vi "输入数据解析.vi"(0 "单个参数补充":dbl, 1 "从板号":dbl=1.0, 2 "主板二维码":string="BNET01", 3 "从板二维码":string="BNET01", 5 "主板引用":refnum<vi>, 7 "从板引用":refnum<vi>, 9 "主板选项":string="三级故障阀值", 11 "枚举":enum16{"主板", "从板"}(ring), 12 "快换":bool caption="快换写入") -> (4 "输出数组":dbl[][](array[numeric]), 6 "数组长度":dbl[](array[numeric]), 8 "循环次数":i32, 10 "命令":u32, 14 "名称":string[](array[string]), 15 "命令序号":u32[](array[numeric]))   [LabVIEW 2013]
panel:
  out "从板信息":T1
  out "主板数据":T2
  out "低位子数组 18":i32[](array[numeric])
  out "低位子数组 17":i32[](array[numeric])
  out "低位子数组 16":i32[](array[numeric])
  out "低位子数组 15":i32[](array[numeric])
  out "低位子数组 14":i32[](array[numeric])
  out "低位子数组 13":i32[](array[numeric])
  out "低位子数组 12":i32[](array[numeric])
  out "低位子数组 11":i32[](array[numeric])
  out "低位子数组 10":i32[](array[numeric])
  out "低位子数组 9":i32[](array[numeric])
  out "低位子数组 8":i32[](array[numeric])
  out "低位子数组 7":i32[](array[numeric])
  out "低位子数组 6":i32[](array[numeric])
  out "低位子数组 5":i32[](array[numeric])
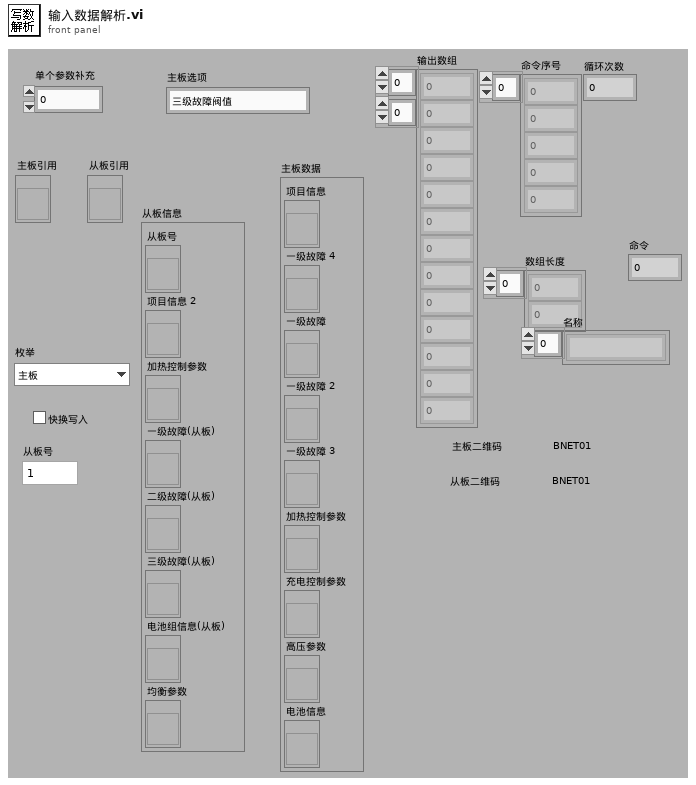
[diagram p1: front panel]
types:
  T1 = cluster{"从板号":refnum<vi>, "项目信息 2":refnum<vi>, "加热控制参数":refnum<vi>, "一级故障(从板)":refnum<vi>, "二级故障(从板)":refnum<vi>, "三级故障(从板)":refnum<vi>, "电池组信息(从板)":refnum<vi>, "均衡参数":refnum<vi>}
  T2 = cluster{"项目信息":refnum<vi>, "一级故障 4":refnum<vi>, "一级故障":refnum<vi>, "一级故障 2":refnum<vi>, "一级故障 3":refnum<vi>, "加热控制参数":refnum<vi>, "充电控制参数":refnum<vi>, "高压参数":refnum<vi>, "电池信息":refnum<vi>}
  T3 = cluster{"电池额定容量(A)":dbl, "使用者":dbl, "电池实际容量(A)":dbl, "车架(牌)号":string, "配置文件版本":string, "SOH(%)":dbl, "SOC(%)":dbl, "产品编号":string, "系统时钟":string}
  T4 = cluster{"总电压过高":dbl, "整组电压不均衡":dbl, "SOC过高":dbl, "单体电压过高":dbl, "总电压过低":dbl, "温度过高":dbl, "温度过低":dbl, "单组电压不均衡":dbl, "整组温度不均衡":dbl, "单组温度不均衡":dbl, "单体电压过低":dbl, "充电电流过高":dbl, "放电电流过高":dbl, "SOC过低":dbl, "内阻过大":dbl, "极柱温度过高":dbl, "SOH过低":dbl}
  T5 = cluster{"风机开启温度":dbl, "风机关闭温度":dbl, "加热开启温度":dbl, "加热关闭温度":dbl, "风机开启温差":dbl, "风机关闭温差":dbl, "加热关闭温差":dbl}
  T6 = cluster{"最大允许单体电压":dbl, "最大允许总电压":dbl, "最小允许单体电压":dbl, "最大允许充电电流":dbl, "最小允许充电电流":dbl, "最大允许充电温度":dbl, "最小允许充电温度":dbl, "电流步长":dbl}
  T7 = cluster{"电池串联":dbl, "电池并联":dbl, "累计放电总安时":dbl, "电池包额定容量":dbl, "电池包额定能量":dbl, "电池包额定总电压":dbl, "累计充电总安时":dbl, "电池充满次数":dbl, "电池放空次数":dbl, "电池充电次数":dbl, "电池生产日期":string, "电池厂家":string, "电池类型":string, "电池包组号":string, "电池包产权标识":string, "电池应用车型":string, "实际容量":dbl}
  T8 = cluster{"电压过高":dbl, "电压过低":dbl, "温度过高":dbl, "温度过低":dbl, "电压不均衡(V)":dbl, "温度不均衡":dbl, "SOC过低":dbl}
  T9 = cluster{"串联数":dbl, "并联数":dbl, "电池厂家":dbl, "电池类型":dbl, "额定能量":dbl, "额定容量":dbl, "实际容量":dbl, "额定总压":dbl, "产权标识":dbl, "应用车型":dbl, "电池包组号":dbl, "SOC":dbl, "充电总安时":dbl, "放电总这时":dbl, "放空次数":dbl, "充满次数":dbl, "充电次数":dbl, "车牌号":string, "生产日期":string, "最大允许单体电压":dbl, "最大允许总电压":dbl, "最大允许温度":dbl, "最小允许温度":dbl, "最大允许充电电流":dbl, "最小允许充电电流":dbl, "最小允许单体电压":dbl, "电流步长":dbl, "电池包序号":dbl}
  T10 = cluster{"充电结束电压(90%)":sgl, "充电结束电压(91%)":sgl, "充电结束电压(92%)":sgl, "充电结束电压(93%)":sgl, "充电结束电压(94%)":sgl, "均衡计算-电压高阀值1级":sgl, "均衡计算-电压高阀值2级":sgl, "均衡计算-电压低阀值1级":sgl, "均衡计算-电压低阀值2级":sgl, "均衡计算-最低电压阀值":sgl, "均衡停止-最低电压阀值":sgl, "均衡计算-电压极差阀值":sgl, "充电结束电压(95%)":sgl, "充电结束电压(96%)":sgl, "充电结束电压(97%)":sgl, "充电结束电压(98%)":sgl, "充电结束电压(99%)":sgl, "充电结束电压(100%)":sgl}
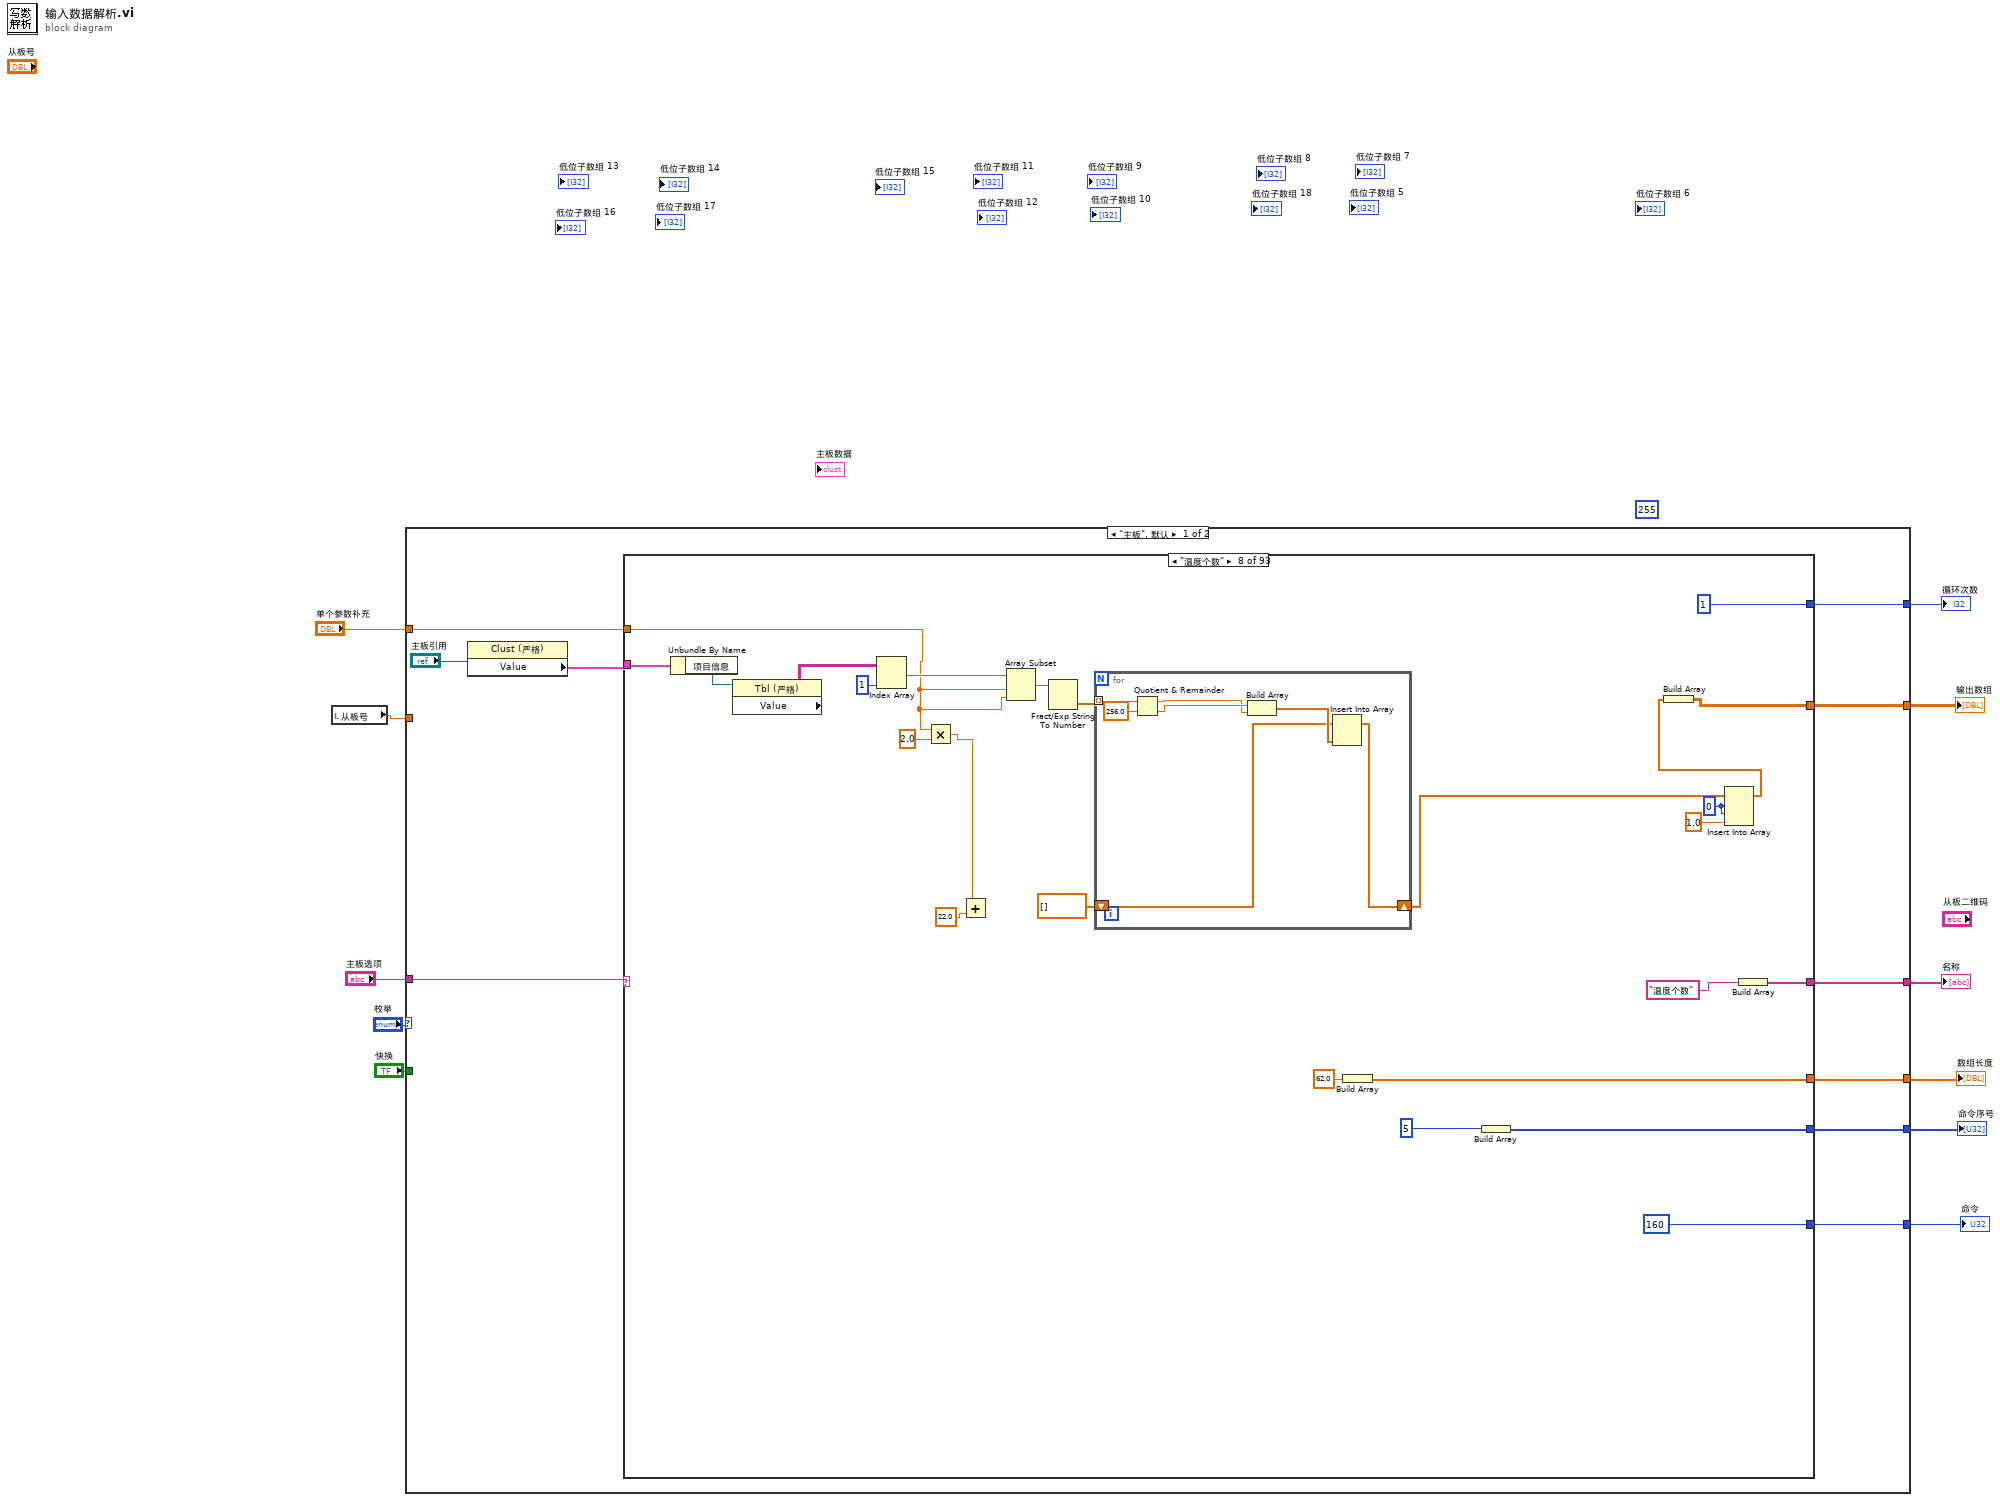
[diagram p0: block diagram]
diagram:
  (unwired) 255 ("高字节1")
  n1 = local read "从板号"() -> (w3:dbl)
  n2 = case shown="\"主板\", 默认" "枚举" {
    tunnel: "主板选项" -> [w21 w14879]
    tunnel: "单个参数补充" -> [w20 w14874]
    tunnel: [w19 w14878] -> w9
    tunnel: [w18 w14876] -> w8
    tunnel: [w17 w14875] -> w7
    tunnel: [w16 w14877] -> w6
    tunnel: "快换" -> [_ w14873]
    tunnel: w3 -> [_ w14872]
    tunnel: [w13 w14869] -> w2
    tunnel: [w12 w14868] -> w1
    frame "主板", Default {
      n3 = property class="Clust (严格)"(reference="主板引用") -> ("Value"=w14:T2)  [unwired: 1 in, 2 out]
      n4 = case shown="\"温度个数\"" w21 {
        tunnel: w20 -> [w29 w290 _ _ w576 w605 w636 w658 w696 _ _ _ _ _ _ _ _ _ _ _ _ _ _ _ _ _ _ _ _ _ _ _ _ _ _ _ _ _ _ _ _ _ _ _ _ _ _ _ _ _ _ _ _ _ _ _ _ _ _ _ _ _ _ _ _ _ _ _ _ _ _ _ _ _ _ _ _ _ _ _ _ _ _ _ _ _ _ _ _ _ _ _ _]
        tunnel: w14 -> [w27 w288 w549 _ w589 w622 w649 w678 w709 w737 w774 w789 w813 _ w845 w863 w870 w1013 w1244 w1475 w1706 w1937 w2168 w2399 w2630 w2861 w3092 w3323 w3554 w3785 w4015 w4245 w4475 w4706 w4937 w5168 w5397 w5626 w5855 w6085 w6315 w6545 w6774 w7003 w7232 w7462 w7692 w7922 w8152 w8382 w8612 w8841 w9070 w9299 w9529 w9759 w9989 w10219 w10449 w10679 w10898 w11116 w11336 w11551 w11766 w11977 w12191 w12405 w12619 w12762 w12921 w12943 w12965 w12987 w13009 w13031 w13053 w13075 w13084 w13159 w13264 w13369 w13474 w13579 w13684 w13789 w13894 w13999 w14151 w14308 w14445 w14582 w14717]
        tunnel: [w28 w289 w536 w555 w571 w615 w642 w664 w690 w725 w745 w780 w796 w820 w836 w851 w874 w1017 w1248 w1479 w1710 w1941 w2172 w2403 w2634 w2865 w3096 w3327 w3558 w3789 w4019 w4249 w4479 w4710 w4941 w5172 w5401 w5630 w5859 w6089 w6319 w6549 w6778 w7007 w7236 w7466 w7696 w7926 w8156 w8386 w8616 w8845 w9074 w9303 w9533 w9763 w9993 w10223 w10453 w10683 w10902 w11120 w11340 w11555 w11770 w11981 w12195 w12409 w12623 w12766 w12925 w12947 w12969 w12991 w13013 w13035 w13057 w13079 w13091 w13166 w13271 w13376 w13481 w13586 w13691 w13796 w13901 w14001 w14153 w14310 w14447 w14584 w14716] -> w19
        tunnel: [w26 w287 w537 w556 w578 w612 w639 w669 w700 w723 w743 w778 w794 w818 w834 w849 u32[] [1] u32[] [1] u32[] [1] u32[] [1] u32[] [2] u32[] [3] u32[] [2] u32[] [3] u32[] [2] u32[] [3] u32[] [1] u32[] [2] u32[] [3] u32[] [1] u32[] [2] u32[] [3] u32[] [1] u32[] [2] u32[] [3] u32[] [1] u32[] [2] u32[] [3] u32[] [1] u32[] [2] u32[] [3] u32[] [1] u32[] [2] u32[] [3] u32[] [1] u32[] [2] u32[] [3] u32[] [1] u32[] [2] u32[] [3] u32[] [1] u32[] [2] u32[] [3] u32[] [1] u32[] [2] u32[] [3] u32[] [1] u32[] [2] u32[] [3] u32[] [1] u32[] [2] u32[] [3] u32[] [1] u32[] [2] u32[] [3] u32[] [1] u32[] [2] u32[] [3] u32[] [2] u32[] [3] u32[] [1] u32[] [1] u32[] [1] u32[] [1] u32[] [1] u32[] [1] u32[] [1] u32[] [1] u32[] [2] u32[] [2] u32[] [2] u32[] [2] u32[] [2] u32[] [2] u32[] [2] u32[] [2] u32[] [2] w14003 w14155 w14312 w14449 w14586 w14718] -> w18
        tunnel: [w25 w286 w538 w557 w580 w614 w641 w671 w702 w724 w744 w779 w795 w819 w835 w850 dbl[] [28.0] dbl[] [28.0] dbl[] [28.0] dbl[] [28.0] dbl[] [28.0] dbl[] [28.0] dbl[] [28.0] dbl[] [28.0] dbl[] [28.0] dbl[] [28.0] dbl[] [28.0] dbl[] [28.0] dbl[] [28.0] dbl[] [28.0] dbl[] [28.0] dbl[] [28.0] dbl[] [28.0] dbl[] [28.0] dbl[] [28.0] dbl[] [28.0] dbl[] [28.0] dbl[] [28.0] dbl[] [28.0] dbl[] [28.0] dbl[] [28.0] dbl[] [28.0] dbl[] [28.0] dbl[] [28.0] dbl[] [28.0] dbl[] [28.0] dbl[] [28.0] dbl[] [28.0] dbl[] [28.0] dbl[] [28.0] dbl[] [28.0] dbl[] [28.0] dbl[] [28.0] dbl[] [28.0] dbl[] [28.0] dbl[] [28.0] dbl[] [28.0] dbl[] [28.0] dbl[] [28.0] dbl[] [28.0] dbl[] [28.0] dbl[] [28.0] dbl[] [28.0] dbl[] [28.0] dbl[] [28.0] dbl[] [28.0] dbl[] [28.0] dbl[] [28.0] dbl[] [28.0] dbl[] [28.0] dbl[] [7.0] dbl[] [7.0] dbl[] [7.0] dbl[] [7.0] dbl[] [7.0] dbl[] [7.0] dbl[] [7.0] dbl[] [7.0] dbl[] [14.0] dbl[] [14.0] dbl[] [14.0] dbl[] [14.0] dbl[] [14.0] dbl[] [14.0] dbl[] [14.0] dbl[] [14.0] dbl[] [14.0] w14004 w14156 w14313 w14450 w14587 w14719] -> w17
        tunnel: [u32 160 ("命令序号") u32 160 ("命令序号") u32 160 ("命令序号") u32 172 ("命令序号") u32 160 ("命令序号") u32 160 ("命令序号") u32 160 ("命令序号") u32 160 ("命令序号") u32 160 ("命令序号") u32 160 ("命令序号") u32 160 ("命令序号") u32 160 ("命令序号") u32 160 ("命令序号") u32 160 ("命令序号") u32 160 ("命令序号") u32 160 ("命令序号") u32 161 ("命令序号") u32 161 ("命令序号") u32 161 ("命令序号") u32 161 ("命令序号") u32 161 ("命令序号") u32 161 ("命令序号") u32 161 ("命令序号") u32 161 ("命令序号") u32 161 ("命令序号") u32 161 ("命令序号") u32 161 ("命令序号") u32 161 ("命令序号") u32 161 ("命令序号") u32 161 ("命令序号") u32 161 ("命令序号") u32 161 ("命令序号") u32 161 ("命令序号") u32 161 ("命令序号") u32 161 ("命令序号") u32 161 ("命令序号") u32 161 ("命令序号") u32 161 ("命令序号") u32 161 ("命令序号") u32 161 ("命令序号") u32 161 ("命令序号") u32 161 ("命令序号") u32 161 ("命令序号") u32 161 ("命令序号") u32 161 ("命令序号") u32 161 ("命令序号") u32 161 ("命令序号") u32 161 ("命令序号") u32 161 ("命令序号") u32 161 ("命令序号") u32 161 ("命令序号") u32 161 ("命令序号") u32 161 ("命令序号") u32 161 ("命令序号") u32 161 ("命令序号") u32 161 ("命令序号") u32 161 ("命令序号") u32 161 ("命令序号") u32 161 ("命令序号") u32 161 ("命令序号") u32 161 ("命令序号") u32 161 ("命令序号") u32 161 ("命令序号") u32 161 ("命令序号") u32 161 ("命令序号") u32 161 ("命令序号") u32 161 ("命令序号") u32 161 ("命令序号") u32 161 ("命令序号") u32 161 ("命令序号") u32 162 ("命令序号") u32 162 ("命令序号") u32 162 ("命令序号") u32 162 ("命令序号") u32 162 ("命令序号") u32 162 ("命令序号") u32 162 ("命令序号") u32 162 ("命令序号") u32 162 ("命令序号") u32 162 ("命令序号") u32 162 ("命令序号") u32 162 ("命令序号") u32 162 ("命令序号") u32 162 ("命令序号") u32 162 ("命令序号") u32 162 ("命令序号") u32 162 ("命令序号") u32 164 ("命令序号") u32 164 ("命令序号") u32 164 ("命令序号") u32 164 ("命令序号") u32 164 ("命令序号") w14720] -> w16
        tunnel: [w23 w284 1 1 1 1 1 1 1 w733 1 1 1 1 1 1 1 1 1 1 1 1 1 1 1 1 1 1 1 1 1 1 1 1 1 1 1 1 1 1 1 1 1 1 1 1 1 1 1 1 1 1 1 1 1 1 1 1 1 1 1 1 1 1 1 1 1 1 1 1 1 1 1 1 1 1 1 1 1 1 1 1 1 1 1 1 1 1 4 1 1 1 _] -> w13
        tunnel: [w22 w283 w543 w559 w568 w601 w632 w660 w686 w721 w741 w776 w791 w815 w832 w847 w865 w1008 w1239 w1470 w1701 w1932 w2163 w2394 w2625 w2856 w3087 w3318 w3549 w3780 w4010 w4240 w4470 w4701 w4932 w5163 w5392 w5621 w5850 w6080 w6310 w6540 w6769 w6998 w7227 w7457 w7687 w7917 w8147 w8377 w8607 w8836 w9065 w9294 w9524 w9754 w9984 w10214 w10444 w10674 w10893 w11111 w11331 w11546 w11761 w11972 w12186 w12400 w12614 w12757 string[] ["加热控制参数"] string[] ["加热控制参数"] string[] ["加热控制参数"] string[] ["加热控制参数"] string[] ["加热控制参数"] string[] ["加热控制参数"] string[] ["加热控制参数"] string[] ["加热控制参数"] string[] ["充电控制参数"] string[] ["充电控制参数"] string[] ["充电控制参数"] string[] ["充电控制参数"] string[] ["充电控制参数"] string[] ["充电控制参数"] string[] ["充电控制参数"] string[] ["充电控制参数"] string[] ["充电控制参数"] string[] ["电池信息1"] w14148 string[] ["电池包组号"] string[] ["充放电安时"] string[] ["电池充放电次数"] _] -> w12
        frame "项目信息", Default {
          w23 = 13
          n5 = for {
            N: w23 -> [_]
            tunnel: w29 -> [w36]
            tunnel: [w35] -> w28 mode=indexing
            tunnel: [w34] -> w26 mode=indexing
            tunnel: w27 -> [w33]
            tunnel: [w32] -> w25 mode=indexing
            tunnel: [w31] -> w22 mode=indexing
            i -> [w30]
            n6 = case shown="1" w30 {
              tunnel: w36 -> [_ w48 w77 w92 w117 w143 w171 _ _ _ _ _ _]
              tunnel: [w43 w51 w71 w91 w115 w141 w164 w222 w234 w241 w247 w268 w282] -> w35
              tunnel: [u32 1 ("命令序号") u32 2 ("命令序号") u32 3 ("命令序号") u32 4 ("命令序号") u32 5 ("命令序号") u32 6 ("命令序号") u32 13 ("命令序号") u32 8 ("命令序号") u32 7 ("命令序号") u32 9 ("命令序号") u32 10 ("命令序号") u32 11 ("命令序号") u32 12 ("命令序号")] -> w34
              tunnel: w33 -> [w41 w52 w76 w93 w118 w142 w170 w203 w230 w238 w248 w265 w278]
              tunnel: [w42 63.0 ("单个参数补充") 20.0 ("单个参数补充") 62.0 ("元素") 62.0 ("元素") 62.0 ("元素") 10.0 ("元素") 8.0 ("单个参数补充") 2.0 ("单个参数补充") w240 8.0 ("单个参数补充") w267 2.0 ("单个参数补充")] -> w32
              tunnel: ["产品编号" "电压个数" "通道电压数" "电压起始值" "温度个数" "温度起始值" "保险位置" "电池额定实际容量" "SOC" "配置文件版本" "参数修改记录" "车牌号" "SOH"] -> w31
              frame 0, Default {
                w42 = 16 ("长度")
                # "产品编号"
                n7 = Unbundle By Name(w41) -> ("一级故障 4"=w40:refnum<vi>)
                n8 = property class="Clust (严格)"(reference=w40) -> ("Value"=w39:T3)  [unwired: 1 in, 2 out]
                n9 = Unbundle By Name(w39) -> ("产品编号"=w38:string)
                n10 = String To Byte Array(string=w38) -> (unsigned byte array=w44:u8[])
                n11 = Array Subset(array=w44, length=w42) -> (w43:u8[])  [unwired: 1 in]
              }
              frame 1 {
                # "电压个数"
                # "电压个数"
                n12 = Unbundle By Name(w52) -> ("项目信息"=w57:refnum<vi>)
                n13 = property class="Tbl (严格)"(reference=w57) -> ("Value"=w56:string[][])  [unwired: 1 in, 2 out]
                n14 = Index Array(array=w56, index (col)=1 ("禁用的索引 (列)")) -> (element=w58:string[])  [unwired: 1 in]
                n15 = Array Subset(array=w58, index=0 ("索引"), length=w48) -> (w61:string[])
                n16 = Fract/Exp String To Number(string=w61) -> (number=w55:dbl[])  [unwired: 4 out]
                n17 = for {
                  tunnel: w55 -> [w70] mode=indexing
                  shift-right: [w65] -> w53
                  shift-left: dbl[] [] -> [w64]
                  n18 = Quotient & Remainder(x=w70, y=256.0) -> (x-y*floor(x/y)=w67:dbl, floor(x/y)=w68:dbl)
                  n19 = Build Array(w68, w67) -> (w66:dbl[])
                  n20 = Insert Into Array(array=w64, new element=w66) -> (w65:dbl[])  [unwired: 1 in]
                }
                n21 = Insert Into Array(array=w53, index=0 ("索引"), new element #1=w48, new element #2=0.0 ("新元素/子数组"), new element #3=1.0 ("新元素/子数组")) -> (w51:dbl[])
              }
              frame 2 {
                # "全部给1"
                n22 = Unbundle By Name(w76) -> ("项目信息"=w81:refnum<vi>)
                n23 = property class="Tbl (严格)"(reference=w81) -> ("Value"=w80:string[][])  [unwired: 1 in, 2 out]
                n24 = Index Array(array=w80, index (col)=1 ("禁用的索引 (列)")) -> (element=w82:string[])  [unwired: 1 in]
                n25 = Increment(x=w77) -> (x+1=w78:dbl)
                n26 = Array Subset(array=w82, index=w78, length=20 ("长度")) -> (w84:string[])
                n27 = Fract/Exp String To Number(string=w84) -> (number=w72:dbl[])  [unwired: 4 out]
                n28 = for {
                  tunnel: [1.0 ("y")] -> w71 mode=indexing
                  tunnel: w72 -> [w86] mode=indexing
                  w87 = 12.0 ("y")
                  n29 = Greater?(x=w86, y=w87) -> (0:w88:bool)
                  n30 = Select(t=w87, s=w88, f=w86) -> ()  [unwired: 1 out]
                }
              }
              frame 3 {
                # "全部给1"
                # "电压起始值"
                n31 = Unbundle By Name(w93) -> ("项目信息"=w100:refnum<vi>)
                n32 = property class="Tbl (严格)"(reference=w100) -> ("Value"=w99:string[][])  [unwired: 1 in, 2 out]
                n33 = Index Array(array=w99, index (col)=1 ("禁用的索引 (列)")) -> (element=w101:string[])  [unwired: 1 in]
                n34 = Add(x=21.0, y=w92) -> (x+y=w96:dbl)
                n35 = Increment(x=w92) -> (x+1=w94:dbl)
                n36 = Array Subset(array=w101, index=w96, length=w94) -> (w103:string[])
                n37 = Fract/Exp String To Number(string=w103) -> (number=w98:dbl[])  [unwired: 4 out]
                n38 = for {
                  tunnel: w98 -> [w111] mode=indexing
                  shift-right: [w108] -> w91
                  shift-left: dbl[] [] -> [w107]
                  n39 = Quotient & Remainder(x=w111, y=256.0) -> ()  [unwired: 2 out]
                  n40 = Build Array(0.0 ("元素"), 1.0 ("元素")) -> (w109:dbl[])
                  n41 = Insert Into Array(array=w107, new element=w109) -> (w108:dbl[])  [unwired: 1 in]
                }
              }
              frame 4 {
                n42 = Unbundle By Name(w118) -> ("项目信息"=w125:refnum<vi>)
                n43 = property class="Tbl (严格)"(reference=w125) -> ("Value"=w124:string[][])  [unwired: 1 in, 2 out]
                n44 = Index Array(array=w124, index (col)=1 ("禁用的索引 (列)")) -> (element=w126:string[])  [unwired: 1 in]
                n45 = Increment(x=w117) -> ()  [unwired: 1 out]
                n46 = Multiply(x=w117, y=2.0) -> (x*y=w122:dbl)
                n47 = Add(x=w122, y=22.0) -> ()  [unwired: 1 out]
                n48 = Array Subset(array=w126, index=w117, length=w117) -> (w128:string[])
                n49 = Fract/Exp String To Number(string=w128) -> (number=w120:dbl[])  [unwired: 4 out]
                n50 = for {
                  tunnel: w120 -> [w138] mode=indexing
                  shift-right: [w133] -> w116
                  shift-left: dbl[] [] -> [w132]
                  n51 = Quotient & Remainder(x=w138, y=256.0) -> (x-y*floor(x/y)=w135:dbl, floor(x/y)=w136:dbl)
                  n52 = Build Array(w136, w135) -> (w134:dbl[])
                  n53 = Insert Into Array(array=w132, new element=w134) -> (w133:dbl[])  [unwired: 1 in]
                }
                n54 = Insert Into Array(array=w116, index=0 ("索引"), new element #1=0.0 ("新元素/子数组"), new element #2=1.0 ("新元素/子数组")) -> (w115:dbl[])
              }
              frame 5 {
                # "全部给1"
                n55 = Unbundle By Name(w142) -> ("项目信息"=w152:refnum<vi>)
                n56 = property class="Tbl (严格)"(reference=w152) -> ("Value"=w151:string[][])  [unwired: 1 in, 2 out]
                n57 = Index Array(array=w151, index (col)=1 ("禁用的索引 (列)")) -> (element=w153:string[])  [unwired: 1 in]
                n58 = Increment(x=w143) -> (x+1=w150:dbl)
                n59 = Multiply(x=w143, y=3.0) -> (x*y=w147:dbl)
                n60 = Add(x=w147, y=23.0) -> (x+y=w149:dbl)
                n61 = Array Subset(array=w153, index=w149, length=w150) -> (w155:string[])
                n62 = Fract/Exp String To Number(string=w155) -> (number=w145:dbl[])  [unwired: 4 out]
                n63 = for {
                  tunnel: w145 -> [w163] mode=indexing
                  shift-right: [w160] -> w141
                  shift-left: dbl[] [] -> [w159]
                  n64 = Quotient & Remainder(x=w163, y=256.0) -> ()  [unwired: 2 out]
                  n65 = Build Array(0.0 ("元素"), 1.0 ("元素")) -> (w161:dbl[])
                  n66 = Insert Into Array(array=w159, new element=w161) -> (w160:dbl[])  [unwired: 1 in]
                }
              }
              frame 6 {
                n67 = Unbundle By Name(w170) -> ("项目信息"=w177:refnum<vi>)
                n68 = property class="Tbl (严格)"(reference=w177) -> ("Value"=w176:string[][])  [unwired: 1 in, 2 out]
                n69 = Multiply(x=w171, y=4.0) -> (x*y=w173:dbl)
                n70 = Add(x=w173, y=24.0) -> (x+y=w175:dbl)
                n71 = Index Array(array=w176, index (col)=1 ("禁用的索引 (列)")) -> (element=w178:string[])  [unwired: 1 in]
                n72 = Array Subset(array=w178, index=w175, length=20 ("长度")) -> (w180:string[])
                n73 = Fract/Exp String To Number(string=w180) -> (number=w166:dbl[])  [unwired: 4 out]
                n74 = for {
                  N: 10 -> [_]
                  tunnel: w166 -> [w191]
                  tunnel: [0] -> w164 mode=indexing
                  i -> [w193]
                  w186 = 4 ("索引")
                  n75 = Multiply(x=w193, y=2) -> (x*y=w190:i32)
                  n76 = Increment(x=w190) -> (x+1=w189:i32)
                  n77 = Index Array(array=w191, index #1=w190, index #2=w189) -> (element #1=w188:dbl, element #2=w187:dbl)
                  n78 = call "二进制解析-8.6.vi"("索引"=w186, "数值"=w188) -> ("低位子数组"=w185:i32[])  [unwired: 1 in, 2 out]
                  n79 = call "二进制解析-8.6.vi"("索引"=w186, "数值"=w187) -> ("低位子数组"=w184:i32[])  [unwired: 1 in, 2 out]
                  n80 = Insert Into Array(array=w185, new element=w184) -> (w183:i32[])  [unwired: 1 in]
                  n81 = call "数值二进制转十进制-8.6.vi"("子数组"=w183) -> ()  [unwired: 4 in, 1 out]
                }
              }
              frame 7 {
                w212 = 256.0 ("y")
                w214 = 256.0 ("y")
                # "电池额定容量,实际容量"
                n82 = Unbundle By Name(w203) -> ("一级故障 4"=w202:refnum<vi>)
                n83 = property class="Clust (严格)"(reference=w202) -> ("Value"=w201:T3)  [unwired: 1 in, 2 out]
                n84 = Unbundle By Name(w201) -> ("电池额定容量(A)"=w199:dbl, "电池实际容量(A)"=w198:dbl)
                n85 = call "输入分辨率计算-EV05.vi"("1字节?"=TRUE, "数值 2"=w198, "数值"=w199, "分辨率"=0.001) -> ("高字节 2"=w196:dbl, "高字节1"=w197:dbl)  [unwired: 1 in, 5 out]
                n86 = Quotient & Remainder(x=w197, y=w214) -> (x-y*floor(x/y)=w218:dbl, floor(x/y)=w220:dbl)
                n87 = Quotient & Remainder(x=w196, y=w212) -> (x-y*floor(x/y)=w205:dbl, floor(x/y)=w209:dbl)
                n88 = Quotient & Remainder(x=w220, y=w214) -> (x-y*floor(x/y)=w217:dbl, floor(x/y)=w219:dbl)
                n89 = Quotient & Remainder(x=w209, y=w212) -> (x-y*floor(x/y)=w206:dbl, floor(x/y)=w210:dbl)
                n90 = Quotient & Remainder(x=w219, y=w214) -> (x-y*floor(x/y)=w216:dbl, floor(x/y)=w215:dbl)
                n91 = Quotient & Remainder(x=w210, y=w212) -> (x-y*floor(x/y)=w207:dbl, floor(x/y)=w211:dbl)
                n92 = Quotient & Remainder(x=w215, y=w214) -> (x-y*floor(x/y)=w213:dbl)  [unwired: 1 out]
                n93 = Quotient & Remainder(x=w211, y=w212) -> (x-y*floor(x/y)=w208:dbl)  [unwired: 1 out]
                n94 = Build Array(w213, w216, w217, w218, w208, w207, w206, w205) -> (w222:dbl[])
              }
              frame 8 {
                # "SOC"
                n95 = Unbundle By Name(w230) -> ("一级故障 4"=w231:refnum<vi>)
                n96 = property class="Clust (严格)"(reference=w231) -> ("Value"=w229:T3)  [unwired: 1 in, 2 out]
                n97 = Unbundle By Name(w229) -> ("SOC(%)"=w227:dbl)
                n98 = call "输入分辨率计算-EV05.vi"("1字节?"=FALSE, "数值"=w227, "分辨率"=0.1) -> ("低字节"=w224:dbl, "高字节1"=w225:dbl)  [unwired: 2 in, 5 out]
                n99 = Build Array(w225, w224) -> (w234:dbl[])
              }
              frame 9 {
                w240 = 8 ("长度")
                # "配置文件版本"
                n100 = Unbundle By Name(w238) -> ("一级故障 4"=w239:refnum<vi>)
                n101 = property class="Clust (严格)"(reference=w239) -> ("Value"=w237:T3)  [unwired: 1 in, 2 out]
                n102 = Unbundle By Name(w237) -> ("配置文件版本"=w236:string)
                n103 = String To Byte Array(string=w236) -> (unsigned byte array=w242:u8[])
                n104 = Array Subset(array=w242, length=w240) -> (w241:u8[])  [unwired: 1 in]
              }
              frame 10 {
                n105 = Unbundle By Name(w248) -> ("一级故障 4"=w254:refnum<vi>)
                n106 = property class="Clust (严格)"(reference=w254) -> ("Value"=w253:T3)  [unwired: 1 in, 2 out]
                n107 = Unbundle By Name(w253) -> ("使用者"=w252:dbl)
                n108 = Quotient & Remainder(x=w252, y=256.0) -> (x-y*floor(x/y)=w249:dbl, floor(x/y)=w250:dbl)
                n109 = call "当前时间解析-8.6.vi"("需要秒？(T)"=TRUE) -> ("年"=w260:u8, "月"=w259:u8, "日"=w258:u8, "时"=w257:u8, "分"=w256:u8, "秒"=w255:u8)  [unwired: 13 out]
                n110 = Build Array(w250, w249, w260, w259, w258, w257, w256, w255) -> (w247:dbl[])
              }
              frame 11 {
                w267 = 8 ("长度")
                # "车牌号"
                n111 = Unbundle By Name(w265) -> ("一级故障 4"=w266:refnum<vi>)
                n112 = property class="Clust (严格)"(reference=w266) -> ("Value"=w264:T3)  [unwired: 1 in, 2 out]
                n113 = Unbundle By Name(w264) -> ("车架(牌)号"=w263:string)
                n114 = String To Byte Array(string=w263) -> (unsigned byte array=w269:u8[])
                n115 = Array Subset(array=w269, length=w267) -> (w268:u8[])  [unwired: 1 in]
              }
              frame 12 {
                # "SOH"
                n116 = Unbundle By Name(w278) -> ("一级故障 4"=w279:refnum<vi>)
                n117 = property class="Clust (严格)"(reference=w279) -> ("Value"=w277:T3)  [unwired: 1 in, 2 out]
                n118 = Unbundle By Name(w277) -> ("SOH(%)"=w276:dbl)
                n119 = call "输入分辨率计算-EV05.vi"("1字节?"=FALSE, "数值"=w276, "分辨率"=0.1) -> ("低字节"=w272:dbl, "高字节1"=w273:dbl)  [unwired: 2 in, 5 out]
                n120 = Build Array(w273, w272) -> (w282:dbl[])
              }
            }
          }
        }
        frame "保险位置" {
          w284 = 1
          n121 = for {
            N: w284 -> [_]
            tunnel: w290 -> [w297]
            tunnel: [w296] -> w289 mode=indexing
            tunnel: [w295] -> w287 mode=indexing
            tunnel: w288 -> [w294]
            tunnel: [w293] -> w286 mode=indexing
            tunnel: [w292] -> w283 mode=indexing
            i -> [w291]
            n122 = case shown="9" w291 {
              tunnel: w297 -> [w305 w331 w357 w368 w390 w417 _ _ _ _ _ _ _]
              tunnel: [w299 w330 w356 w367 w388 w415 w444 w475 w487 w494 w500 w521 w535] -> w296
              tunnel: [u32 13 ("命令序号") u32 2 ("命令序号") u32 3 ("命令序号") u32 4 ("命令序号") u32 5 ("命令序号") u32 6 ("命令序号") u32 1 ("命令序号") u32 8 ("命令序号") u32 7 ("命令序号") u32 9 ("命令序号") u32 10 ("命令序号") u32 11 ("命令序号") u32 12 ("命令序号")] -> w295
              tunnel: w294 -> [w304 w332 w355 w369 w389 w416 w442 w456 w483 w491 w501 w518 w531]
              tunnel: [10.0 ("元素") 63.0 ("单个参数补充") 20.0 ("单个参数补充") 62.0 ("元素") 62.0 ("元素") 62.0 ("元素") w443 8.0 ("单个参数补充") 2.0 ("单个参数补充") w493 8.0 ("单个参数补充") w520 2.0 ("单个参数补充")] -> w293
              tunnel: ["保险位置" "电压个数" "通道电压数" "电压起始值" "温度个数" "温度起始值" "产品编号" "电池额定实际容量" "SOC" "配置文件版本" "参数修改记录" "车牌号" "SOH"] -> w292
              frame 0, Default {
                n123 = Unbundle By Name(w304) -> ("项目信息"=w311:refnum<vi>)
                n124 = property class="Tbl (严格)"(reference=w311) -> ("Value"=w310:string[][])  [unwired: 1 in, 2 out]
                n125 = Multiply(x=w305, y=4.0) -> (x*y=w307:dbl)
                n126 = Add(x=w307, y=24.0) -> (x+y=w309:dbl)
                n127 = Index Array(array=w310, index (col)=1 ("禁用的索引 (列)")) -> (element=w312:string[])  [unwired: 1 in]
                n128 = Array Subset(array=w312, index=w309, length=20 ("长度")) -> (w314:string[])
                n129 = Fract/Exp String To Number(string=w314) -> (number=w300:dbl[])  [unwired: 4 out]
                n130 = for {
                  N: 10 -> [_]
                  tunnel: w300 -> [w325]
                  tunnel: [w316] -> w299 mode=indexing
                  i -> [w327]
                  w320 = 4 ("索引")
                  n131 = Multiply(x=w327, y=2) -> (x*y=w324:i32)
                  n132 = Increment(x=w324) -> (x+1=w323:i32)
                  n133 = Index Array(array=w325, index #1=w324, index #2=w323) -> (element #1=w322:dbl, element #2=w321:dbl)
                  n134 = call "二进制解析-8.6.vi"("索引"=w320, "数值"=w322) -> ("低位子数组"=w319:i32[])  [unwired: 1 in, 2 out]
                  n135 = call "二进制解析-8.6.vi"("索引"=w320, "数值"=w321) -> ("低位子数组"=w318:i32[])  [unwired: 1 in, 2 out]
                  n136 = Insert Into Array(array=w319, new element=w318) -> (w317:i32[])  [unwired: 1 in]
                  n137 = call "数值二进制转十进制-8.6.vi"("子数组"=w317) -> ("十进制数值"=w316:i32)  [unwired: 4 in]
                }
              }
              frame 1 {
                # "电压个数"
                # "电压个数"
                n138 = Unbundle By Name(w332) -> ("项目信息"=w338:refnum<vi>)
                n139 = property class="Tbl (严格)"(reference=w338) -> ("Value"=w337:string[][])  [unwired: 1 in, 2 out]
                n140 = Index Array(array=w337, index (col)=1 ("禁用的索引 (列)")) -> (element=w339:string[])  [unwired: 1 in]
                n141 = Increment(x=w331) -> (x+1=w333:dbl)
                n142 = Array Subset(array=w339, index=0 ("索引"), length=w333) -> (w342:string[])
                n143 = Fract/Exp String To Number(string=w342) -> (number=w336:dbl[])  [unwired: 4 out]
                n144 = for {
                  tunnel: w336 -> [w351] mode=indexing
                  shift-right: [w346] -> w334
                  shift-left: dbl[] [] -> [w345]
                  n145 = Quotient & Remainder(x=w351, y=256.0) -> (x-y*floor(x/y)=w348:dbl, floor(x/y)=w349:dbl)
                  n146 = Build Array(w349, w348) -> (w347:dbl[])
                  n147 = Insert Into Array(array=w345, new element=w347) -> (w346:dbl[])  [unwired: 1 in]
                }
                n148 = Insert Into Array(array=w334, index=0 ("索引"), new element=w331) -> (w330:dbl[])
              }
              frame 2 {
                n149 = Unbundle By Name(w355) -> ("项目信息"=w361:refnum<vi>)
                n150 = property class="Tbl (严格)"(reference=w361) -> ("Value"=w360:string[][])  [unwired: 1 in, 2 out]
                n151 = Index Array(array=w360, index (col)=1 ("禁用的索引 (列)")) -> (element=w362:string[])  [unwired: 1 in]
                n152 = Increment(x=w357) -> (x+1=w358:dbl)
                n153 = Array Subset(array=w362, index=w358, length=20 ("长度")) -> (w364:string[])
                n154 = Fract/Exp String To Number(string=w364) -> (number=w356:dbl[])  [unwired: 4 out]
              }
              frame 3 {
                # "电压起始值"
                n155 = Unbundle By Name(w369) -> ("项目信息"=w376:refnum<vi>)
                n156 = property class="Tbl (严格)"(reference=w376) -> ("Value"=w375:string[][])  [unwired: 1 in, 2 out]
                n157 = Index Array(array=w375, index (col)=1 ("禁用的索引 (列)")) -> (element=w377:string[])  [unwired: 1 in]
                n158 = Add(x=21.0, y=w368) -> (x+y=w372:dbl)
                n159 = Increment(x=w368) -> (x+1=w370:dbl)
                n160 = Array Subset(array=w377, index=w372, length=w370) -> (w379:string[])
                n161 = Fract/Exp String To Number(string=w379) -> (number=w374:dbl[])  [unwired: 4 out]
                n162 = for {
                  tunnel: w374 -> [w387] mode=indexing
                  shift-right: [w382] -> w367
                  shift-left: dbl[] [] -> [w381]
                  n163 = Quotient & Remainder(x=w387, y=256.0) -> (x-y*floor(x/y)=w384:dbl, floor(x/y)=w385:dbl)
                  n164 = Build Array(w385, w384) -> (w383:dbl[])
                  n165 = Insert Into Array(array=w381, new element=w383) -> (w382:dbl[])  [unwired: 1 in]
                }
              }
              frame 4 {
                n166 = Unbundle By Name(w389) -> ("项目信息"=w399:refnum<vi>)
                n167 = property class="Tbl (严格)"(reference=w399) -> ("Value"=w398:string[][])  [unwired: 1 in, 2 out]
                n168 = Index Array(array=w398, index (col)=1 ("禁用的索引 (列)")) -> (element=w400:string[])  [unwired: 1 in]
                n169 = Increment(x=w390) -> (x+1=w397:dbl)
                n170 = Multiply(x=w390, y=2.0) -> (x*y=w394:dbl)
                n171 = Add(x=w394, y=22.0) -> (x+y=w396:dbl)
                n172 = Array Subset(array=w400, index=w396, length=w397) -> (w402:string[])
                n173 = Fract/Exp String To Number(string=w402) -> (number=w392:dbl[])  [unwired: 4 out]
                n174 = for {
                  tunnel: w392 -> [w412] mode=indexing
                  shift-right: [w407] -> w388
                  shift-left: dbl[] [] -> [w406]
                  n175 = Quotient & Remainder(x=w412, y=256.0) -> (x-y*floor(x/y)=w409:dbl, floor(x/y)=w410:dbl)
                  n176 = Build Array(w410, w409) -> (w408:dbl[])
                  n177 = Insert Into Array(array=w406, new element=w408) -> (w407:dbl[])  [unwired: 1 in]
                }
              }
              frame 5 {
                n178 = Unbundle By Name(w416) -> ("项目信息"=w426:refnum<vi>)
                n179 = property class="Tbl (严格)"(reference=w426) -> ("Value"=w425:string[][])  [unwired: 1 in, 2 out]
                n180 = Index Array(array=w425, index (col)=1 ("禁用的索引 (列)")) -> (element=w427:string[])  [unwired: 1 in]
                n181 = Increment(x=w417) -> (x+1=w424:dbl)
                n182 = Multiply(x=w417, y=3.0) -> (x*y=w421:dbl)
                n183 = Add(x=w421, y=23.0) -> (x+y=w423:dbl)
                n184 = Array Subset(array=w427, index=w423, length=w424) -> (w429:string[])
                n185 = Fract/Exp String To Number(string=w429) -> (number=w419:dbl[])  [unwired: 4 out]
                n186 = for {
                  tunnel: w419 -> [w437] mode=indexing
                  shift-right: [w432] -> w415
                  shift-left: dbl[] [] -> [w431]
                  n187 = Quotient & Remainder(x=w437, y=256.0) -> (x-y*floor(x/y)=w434:dbl, floor(x/y)=w435:dbl)
                  n188 = Build Array(w435, w434) -> (w433:dbl[])
                  n189 = Insert Into Array(array=w431, new element=w433) -> (w432:dbl[])  [unwired: 1 in]
                }
              }
              frame 12 {
                w443 = 16 ("长度")
                # "产品编号"
                n190 = Unbundle By Name(w442) -> ("一级故障 4"=w441:refnum<vi>)
                n191 = property class="Clust (严格)"(reference=w441) -> ("Value"=w440:T3)  [unwired: 1 in, 2 out]
                n192 = Unbundle By Name(w440) -> ("产品编号"=w439:string)
                n193 = String To Byte Array(string=w439) -> (unsigned byte array=w445:u8[])
                n194 = Array Subset(array=w445, length=w443) -> (w444:u8[])  [unwired: 1 in]
              }
              frame 6 {
                w465 = 256.0 ("y")
                w467 = 256.0 ("y")
                # "电池额定容量,实际容量"
                n195 = Unbundle By Name(w456) -> ("一级故障 4"=w455:refnum<vi>)
                n196 = property class="Clust (严格)"(reference=w455) -> ("Value"=w454:T3)  [unwired: 1 in, 2 out]
                n197 = Unbundle By Name(w454) -> ("电池额定容量(A)"=w452:dbl, "电池实际容量(A)"=w451:dbl)
                n198 = call "输入分辨率计算-EV05.vi"("1字节?"=TRUE, "数值 2"=w451, "数值"=w452, "分辨率"=0.1) -> ("高字节 2"=w449:dbl, "高字节1"=w450:dbl)  [unwired: 1 in, 5 out]
                n199 = Quotient & Remainder(x=w450, y=w467) -> (x-y*floor(x/y)=w471:dbl, floor(x/y)=w473:dbl)
                n200 = Quotient & Remainder(x=w449, y=w465) -> (x-y*floor(x/y)=w458:dbl, floor(x/y)=w462:dbl)
                n201 = Quotient & Remainder(x=w473, y=w467) -> (x-y*floor(x/y)=w470:dbl, floor(x/y)=w472:dbl)
                n202 = Quotient & Remainder(x=w462, y=w465) -> (x-y*floor(x/y)=w459:dbl, floor(x/y)=w463:dbl)
                n203 = Quotient & Remainder(x=w472, y=w467) -> (x-y*floor(x/y)=w469:dbl, floor(x/y)=w468:dbl)
                n204 = Quotient & Remainder(x=w463, y=w465) -> (x-y*floor(x/y)=w460:dbl, floor(x/y)=w464:dbl)
                n205 = Quotient & Remainder(x=w468, y=w467) -> (x-y*floor(x/y)=w466:dbl)  [unwired: 1 out]
                n206 = Quotient & Remainder(x=w464, y=w465) -> (x-y*floor(x/y)=w461:dbl)  [unwired: 1 out]
                n207 = Build Array(w466, w469, w470, w471, w461, w460, w459, w458) -> (w475:dbl[])
              }
              frame 7 {
                # "SOC"
                n208 = Unbundle By Name(w483) -> ("一级故障 4"=w484:refnum<vi>)
                n209 = property class="Clust (严格)"(reference=w484) -> ("Value"=w482:T3)  [unwired: 1 in, 2 out]
                n210 = Unbundle By Name(w482) -> ("SOC(%)"=w480:dbl)
                n211 = call "输入分辨率计算-EV05.vi"("1字节?"=FALSE, "数值"=w480, "分辨率"=0.1) -> ("低字节"=w477:dbl, "高字节1"=w478:dbl)  [unwired: 2 in, 5 out]
                n212 = Build Array(w478, w477) -> (w487:dbl[])
              }
              frame 8 {
                w493 = 8 ("长度")
                # "配置文件版本"
                n213 = Unbundle By Name(w491) -> ("一级故障 4"=w492:refnum<vi>)
                n214 = property class="Clust (严格)"(reference=w492) -> ("Value"=w490:T3)  [unwired: 1 in, 2 out]
                n215 = Unbundle By Name(w490) -> ("配置文件版本"=w489:string)
                n216 = String To Byte Array(string=w489) -> (unsigned byte array=w495:u8[])
                n217 = Array Subset(array=w495, length=w493) -> (w494:u8[])  [unwired: 1 in]
              }
              frame 9 {
                n218 = Unbundle By Name(w501) -> ("一级故障 4"=w507:refnum<vi>)
                n219 = property class="Clust (严格)"(reference=w507) -> ("Value"=w506:T3)  [unwired: 1 in, 2 out]
                n220 = Unbundle By Name(w506) -> ("使用者"=w505:dbl)
                n221 = Quotient & Remainder(x=w505, y=256.0) -> (x-y*floor(x/y)=w502:dbl, floor(x/y)=w503:dbl)
                n222 = call "当前时间解析-8.6.vi"("需要秒？(T)"=TRUE) -> ("年"=w513:u8, "月"=w512:u8, "日"=w511:u8, "时"=w510:u8, "分"=w509:u8, "秒"=w508:u8)  [unwired: 13 out]
                n223 = Build Array(w503, w502, w513, w512, w511, w510, w509, w508) -> (w500:dbl[])
              }
              frame 10 {
                w520 = 8 ("长度")
                # "车牌号"
                n224 = Unbundle By Name(w518) -> ("一级故障 4"=w519:refnum<vi>)
                n225 = property class="Clust (严格)"(reference=w519) -> ("Value"=w517:T3)  [unwired: 1 in, 2 out]
                n226 = Unbundle By Name(w517) -> ("车架(牌)号"=w516:string)
                n227 = String To Byte Array(string=w516) -> (unsigned byte array=w522:u8[])
                n228 = Array Subset(array=w522, length=w520) -> (w521:u8[])  [unwired: 1 in]
              }
              frame 11 {
                # "SOH"
                n229 = Unbundle By Name(w531) -> ("一级故障 4"=w532:refnum<vi>)
                n230 = property class="Clust (严格)"(reference=w532) -> ("Value"=w530:T3)  [unwired: 1 in, 2 out]
                n231 = Unbundle By Name(w530) -> ("SOH(%)"=w529:dbl)
                n232 = call "输入分辨率计算-EV05.vi"("1字节?"=FALSE, "数值"=w529, "分辨率"=0.1) -> ("低字节"=w525:dbl, "高字节1"=w526:dbl)  [unwired: 2 in, 5 out]
                n233 = Build Array(w526, w525) -> (w535:dbl[])
              }
            }
          }
        }
        frame "产品编号" {
          w547 = 16 ("长度")
          # "产品编号"
          n234 = Unbundle By Name(w549) -> ("一级故障 4"=w541:refnum<vi>)
          n235 = property class="Clust (严格)"(reference=w541) -> ("Value"=w540:T3)  [unwired: 1 in, 2 out]
          n236 = Unbundle By Name(w540) -> ("产品编号"=w539:string)
          n237 = String To Byte Array(string=w539) -> (unsigned byte array=w542:u8[])
          n238 = Array Subset(array=w542, length=w547) -> (w550:u8[])  [unwired: 1 in]
          n239 = Build Array(w550) -> (w536:u8[][])
          n240 = Build Array(w547) -> (w538:i32[])
          n241 = Build Array(u32 1 ("命令序号")) -> (w537:u32[])
          n242 = Build Array("产品编号") -> (w543:string[])
        }
        frame "二维码" {
          w563 = 30 ("长度")
          # "产品编号"
          n243 = local read "主板二维码"() -> (w554:string)
          n244 = Search and Replace String(input string=w554, search string="BNET" ("搜索字符串"), replace string="") -> (result string=w551:string)  [unwired: 5 in, 3 out]
          n245 = String To Byte Array(string=w551) -> (unsigned byte array=w558:u8[])
          n246 = Array Subset(array=w558, length=w563) -> (w565:u8[])  [unwired: 1 in]
          n247 = Build Array(w565) -> (w555:u8[][])
          n248 = Build Array(w563) -> (w557:i32[])
          n249 = Build Array(u32 1 ("命令序号")) -> (w556:u32[])
          n250 = Build Array("写二维码") -> (w559:string[])
        }
        frame "电压个数" {
          # "电压个数"
          n251 = Unbundle By Name(w589) -> ("项目信息"=w582:refnum<vi>)
          n252 = property class="Tbl (严格)"(reference=w582) -> ("Value"=w581:string[][])  [unwired: 1 in, 2 out]
          n253 = disable-structure shown="禁用" {
            disable-tunnel: w576 -> [w592 w593]
            disable-tunnel: [w591 w593] -> w572
            frame Disabled {
              n254 = Increment(x=w592) -> (x+1=w591:dbl)
            }
            frame Enabled {
            }
          }
          n255 = Index Array(array=w581, index (col)=1 ("禁用的索引 (列)")) -> (element=w583:string[])  [unwired: 1 in]
          n256 = Array Subset(array=w583, index=0 ("索引"), length=w572) -> (w586:string[])
          n257 = Fract/Exp String To Number(string=w586) -> (number=w575:dbl[])  [unwired: 4 out]
          n258 = for {
            tunnel: w575 -> [w600] mode=indexing
            shift-right: [w595] -> w573
            shift-left: dbl[] [] -> [w594]
            n259 = Quotient & Remainder(x=w600, y=256.0) -> (x-y*floor(x/y)=w597:dbl, floor(x/y)=w598:dbl)
            n260 = Build Array(w598, w597) -> (w596:dbl[])
            n261 = Insert Into Array(array=w594, new element=w596) -> (w595:dbl[])  [unwired: 1 in]
          }
          n262 = Build Array(63.0 ("元素")) -> (w580:dbl[])
          n263 = Build Array(u32 2 ("命令序号")) -> (w578:u32[])
          n264 = Insert Into Array(array=w573, index=0 ("索引"), new element #1=w576, new element #2=0.0 ("新元素/子数组"), new element #3=1.0 ("新元素/子数组")) -> (w590:dbl[])
          n265 = Build Array(w590) -> (w571:dbl[][])
          n266 = Build Array("电压个数") -> (w568:string[])
        }
        frame "电压起始值" {
          n267 = Unbundle By Name(w622) -> ("项目信息"=w617:refnum<vi>)
          n268 = property class="Tbl (严格)"(reference=w617) -> ("Value"=w616:string[][])  [unwired: 1 in, 2 out]
          n269 = Index Array(array=w616, index (col)=1 ("禁用的索引 (列)")) -> (element=w618:string[])  [unwired: 1 in]
          n270 = Add(x=21.0, y=w605) -> (x+y=w607:dbl)
          n271 = Increment(x=w605) -> (x+1=w604:dbl)
          n272 = Array Subset(array=w618, index=w607, length=w604) -> (w620:string[])
          n273 = Fract/Exp String To Number(string=w620) -> (number=w610:dbl[])  [unwired: 4 out]
          n274 = for {
            tunnel: w610 -> [w629] mode=indexing
            shift-right: [w624] -> w608
            shift-left: dbl[] [] -> [w623]
            n275 = Quotient & Remainder(x=w629, y=256.0) -> (x-y*floor(x/y)=w626:dbl, floor(x/y)=w627:dbl)
            n276 = Build Array(w627, w626) -> (w625:dbl[])
            n277 = Insert Into Array(array=w623, new element=w625) -> (w624:dbl[])  [unwired: 1 in]
          }
          n278 = Build Array(62.0 ("元素")) -> (w614:dbl[])
          n279 = Build Array(u32 4 ("命令序号")) -> (w612:u32[])
          n280 = Build Array(w608) -> (w615:dbl[][])
          n281 = Build Array("电压起始值") -> (w601:string[])
        }
        frame "通道电压数" {
          n282 = Unbundle By Name(w649) -> ("项目信息"=w644:refnum<vi>)
          n283 = property class="Tbl (严格)"(reference=w644) -> ("Value"=w643:string[][])  [unwired: 1 in, 2 out]
          n284 = Index Array(array=w643, index (col)=1 ("禁用的索引 (列)")) -> (element=w645:string[])  [unwired: 1 in]
          n285 = Increment(x=w636) -> (x+1=w635:dbl)
          n286 = Array Subset(array=w645, index=w635, length=20 ("长度")) -> (w647:string[])
          n287 = Fract/Exp String To Number(string=w647) -> (number=w631:dbl[])  [unwired: 4 out]
          n288 = for {
            tunnel: w631 -> [w651] mode=indexing
            tunnel: [w650] -> w630 mode=indexing
            w652 = 12.0 ("y")
            n289 = Greater?(x=w651, y=w652) -> (0:w653:bool)
            n290 = Select(t=w652, s=w653, f=w651) -> (s? t:f=w650:dbl)
          }
          n291 = Build Array(w630) -> (w642:dbl[][])
          n292 = Build Array(20.0 ("元素")) -> (w641:dbl[])
          n293 = Build Array(u32 3 ("命令序号")) -> (w639:u32[])
          n294 = Build Array("通道电压数") -> (w632:string[])
        }
        frame "温度个数" {
          w657 = 0 ("索引")
          n295 = Unbundle By Name(w678) -> ("项目信息"=w673:refnum<vi>)
          n296 = property class="Tbl (严格)"(reference=w673) -> ("Value"=w672:string[][])  [unwired: 1 in, 2 out]
          n297 = Index Array(array=w672, index (col)=1 ("禁用的索引 (列)")) -> (element=w674:string[])  [unwired: 1 in]
          n298 = Multiply(x=w658, y=2.0) -> (x*y=w659:dbl)
          n299 = Add(x=w659, y=22.0) -> ()  [unwired: 1 out]
          n300 = Array Subset(array=w674, index=w658, length=w658) -> (w676:string[])
          n301 = Fract/Exp String To Number(string=w676) -> (number=w665:dbl[])  [unwired: 4 out]
          n302 = for {
            tunnel: w665 -> [w685] mode=indexing
            shift-right: [w680] -> w655
            shift-left: dbl[] [] -> [w679]
            n303 = Quotient & Remainder(x=w685, y=256.0) -> (x-y*floor(x/y)=w682:dbl, floor(x/y)=w683:dbl)
            n304 = Build Array(w683, w682) -> (w681:dbl[])
            n305 = Insert Into Array(array=w679, new element=w681) -> (w680:dbl[])  [unwired: 1 in]
          }
          n306 = Build Array(62.0 ("元素")) -> (w671:dbl[])
